vi "R5SetCalibrateConstant.vi"(0 "Signal":string, 1 "LabVIEW Web Service Request":refnum<class "Web Request.lvclass">, 5 "Write":bool, 7 "ReactorNo":i32=1, 9 "Slope":dbl, 11 "Intercept":dbl) -> (4 "Status":string[](array[string]), 8 "OldSlope":dbl, 10 "OldIntercept":dbl, 14 "NewIntercept":dbl, 15 "NewSlope":dbl)   [LabVIEW 2016]
uses:
  <vilib>/wsapi/Web Request.lvclass
  <resource>/objmgr/ni.var.rc
panel:
  in  "cRIONo":i32=1
  # "Use the Web Service Request input terminal to call the VIs on the Web Services palette. Do not remove it from the connector pane unless you don't need access to the palette."
  # "Each additional control wired to the connector pane will be available as an input in the URL. To include an indicator in terminal-mode output (the default setting), it must also be wired to the connector pane."
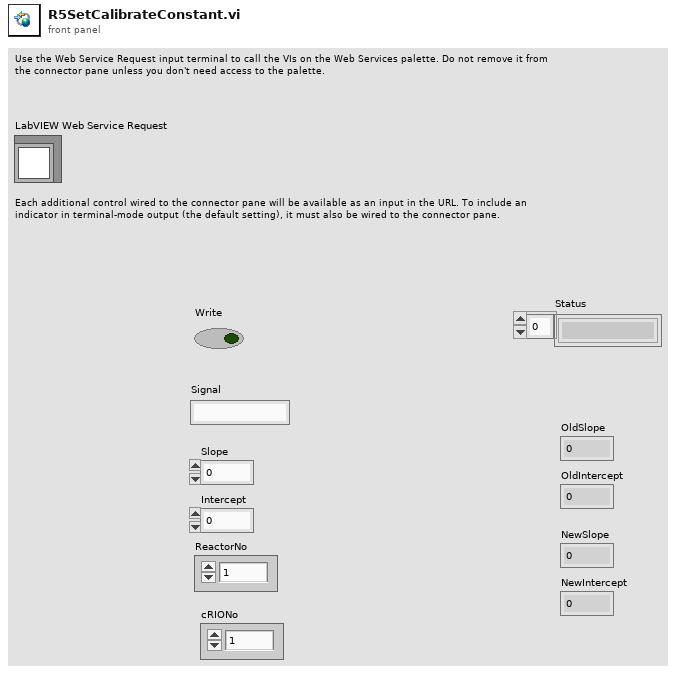
[diagram p1: front panel]
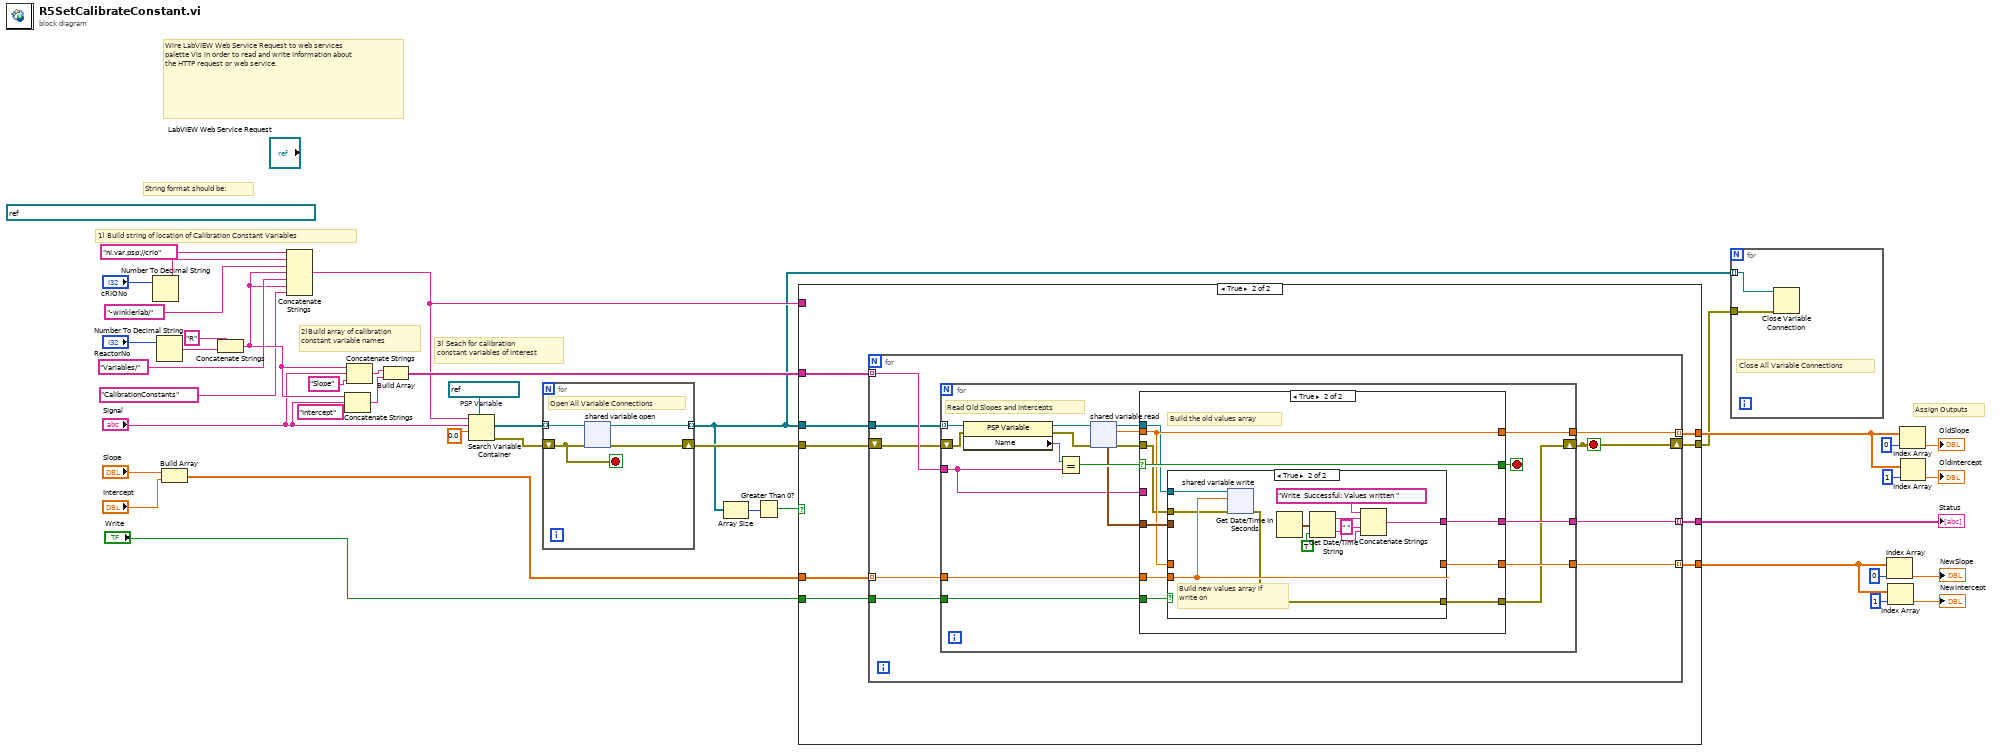
[diagram p0: block diagram]
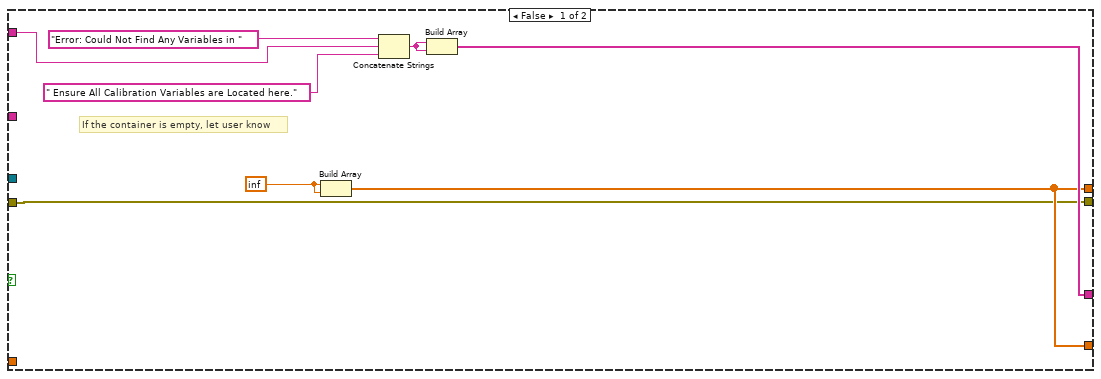
[diagram p2: hidden frame]
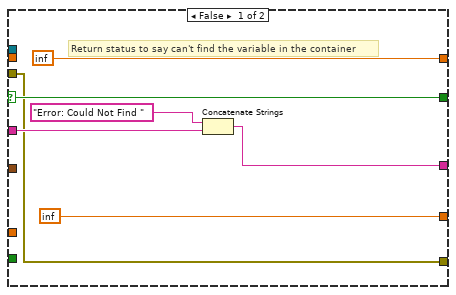
[diagram p3: hidden frame]
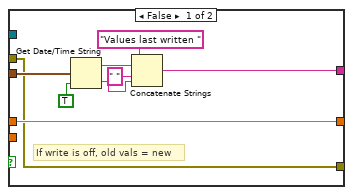
[diagram p4: hidden frame]
diagram:
  w25 = refnum<k21> refnum  # PSP Variable
  (unwired) refnum<k21> "ni.var.psp://crio1-winklerlab/R1Variables/R1CalibrationConstants" ("container refnum in")
  # "Assign Outputs"
  # "3) Seach for calibration \nconstant variables of interest"
  # "2)Build array of calibration \nconstant variable names"
  # "1) Build string of location of Calibration Constant Variables"
  # "String format should be:"
  # "Wire LabVIEW Web Service Request to web services palette VIs in order to read and write information about the HTTP request or web service."
  n1 = Number To Decimal String(number="cRIONo") -> (decimal integer string=w30:string)  [unwired: 1 in]
  n2 = Number To Decimal String(number="ReactorNo") -> (decimal integer string=w38:string)  [unwired: 1 in]
  n3 = Build Array("Slope", "Intercept") -> (w23:dbl[])
  n4 = Concatenate Strings("R" ("string"), w38) -> (w27:string)
  n5 = Concatenate Strings("ni.var.psp://crio" ("string"), w30, "-winklerlab/" ("string"), w27, "Variables/" ("string"), w27, "CalibrationConstants" ("string")) -> (w7:string)
  n6 = Concatenate Strings(w27, "Signal", "Intercept") -> (w36:string)
  n7 = Concatenate Strings(w27, "Signal", "Slope") -> (w37:string)
  n8 = Build Array(w37, w36) -> (w35:string[])
  n9 = Search Variable Container(7:w25, 9:0.0, 10:"Signal", 11:w7) -> (0:w11:errorcluster, 2:w12:refnum<k21>[])  [unwired: 2 in, 1 out]
  n10 = for {
    tunnel: w12 -> [w45] mode=indexing
    shift-right: [w44] -> w10
    shift-left: w11 -> [w42]
    tunnel: [w43] -> w1 mode=indexing
    stop <- w42 stop-if-true
    # "Open All Variable Connections"
    n11 = shared-variable-open(w45, w42) -> (w43:refnum<k21>, w44:errorcluster)  [unwired: 1 in]
  }
  n12 = Array Size(array=w1) -> (size(s)=w9:i32)
  n13 = Greater Than 0?(x=w9) -> (x > 0?=w8:bool)
  n14 = case shown="True" w8 {
    tunnel: w35 -> [_ w62]
    tunnel: "Write" -> [_ w61]
    tunnel: w23 -> [_ w60]
    tunnel: [w48 w59] -> w20
    tunnel: [w48 w58] -> w15
    tunnel: [w49 w57] -> w6
    tunnel: w1 -> [_ w56]
    tunnel: w10 -> [w46 w54]
    tunnel: w7 -> [w52 _]
    tunnel: [w46 w55] -> w2
    frame False {
      w50 = inf
      # "If the container is empty, let user know"
      n15 = Build Array(w50, w50) -> (w48:dbl[])
      n16 = Concatenate Strings("Error: Could Not Find Any Variables in " ("string"), w52, " Ensure All Calibration Variables are Located here." ("string")) -> (w51:string)
      n17 = Build Array(w51, w51) -> (w49:string[])
    }
    frame True {
      n18 = for {
        tunnel: w62 -> [w71] mode=indexing
        tunnel: w56 -> [w65]
        tunnel: w61 -> [w70]
        tunnel: w60 -> [w67] mode=indexing
        tunnel: [w69] -> w59 mode=indexing
        tunnel: [w68] -> w58 mode=indexing
        tunnel: [w66] -> w57 mode=indexing
        shift-right: [w64] -> w55
        shift-left: w54 -> [w63]
        stop <- w64 stop-if-true
        n19 = for {
          tunnel: w65 -> [w77] mode=indexing
          tunnel: w71 -> [w80]
          tunnel: w70 -> [w83]
          tunnel: [w85] -> w69
          tunnel: [w82] -> w68
          tunnel: [w81] -> w66
          tunnel: w67 -> [w79]
          shift-right: [w72] -> w64
          shift-left: w63 -> [w75]
          stop <- w78 stop-if-true
          # "Read Old Slopes and Intercepts"
          n20 = property class="PSP Variable"(reference=w77, error in=w75) -> (reference out=w76:refnum<k21>, error out=w74:errorcluster, "Name"=w73:string)
          n21 = Equal?(x=w73, y=w80) -> (x = y?=w86:bool)
          n22 = shared-variable-read(w76, w74) -> (w89:refnum<k21>, w87:errorcluster, w88:dbl, w84:timestamp)
          n23 = case shown="True" w86 {
            selector: w86 -> [w96 w106]
            tunnel: w89 -> [_ w99]
            tunnel: w88 -> [_ w103]
            tunnel: w87 -> [w90 w98]
            tunnel: [w96 w106] -> w78
            tunnel: [inf w103] -> w85
            tunnel: w84 -> [_ w105]
            tunnel: w83 -> [_ w104]
            tunnel: [inf w102] -> w82
            tunnel: [w92 w101] -> w81
            tunnel: w80 -> [w93 _]
            tunnel: w79 -> [_ w100]
            tunnel: [w90 w97] -> w72
            frame False {
              # "Return status to say can't find the variable in the container"
              n24 = Concatenate Strings("Error: Could Not Find " ("string"), w93) -> (w92:string)
            }
            frame True {
              # "Build the old values array"
              n25 = case shown="True" w104 {
                tunnel: w105 -> [w114 _]
                tunnel: [w110 w120] -> w101
                tunnel: w103 -> [w108 _]
                tunnel: [w108 w118] -> w102
                tunnel: w100 -> [_ w118]
                tunnel: w99 -> [_ w119]
                tunnel: w98 -> [w107 w117]
                tunnel: [w107 w116] -> w97
                frame False {
                  # "If write is off, old vals = new"
                  n26 = Get Date/Time String(seconds (now)=w114, want seconds? (F)=TRUE) -> (date string=w113:string, time string=w111:string)  [unwired: 1 in]
                  n27 = Concatenate Strings("Values last written " ("string"), w113, " " ("string"), w111) -> (w110:string)
                }
                frame True {
                  # "Build new values array if \nwrite on"
                  n28 = shared-variable-write(w119, w117, w118) -> (w116:errorcluster)  [unwired: 1 out]
                  n29 = Get Date/Time In Seconds() -> (seconds since 1Jan1904=w121:timestamp)
                  n30 = Get Date/Time String(seconds (now)=w121, want seconds? (F)=TRUE) -> (date string=w123:string, time string=w125:string)  [unwired: 1 in]
                  n31 = Concatenate Strings("Write  Successful: Values written " ("string"), w123, " " ("string"), w125) -> (w120:string)
                }
              }
            }
          }
        }
      }
    }
  }
  "Status" <- w6
  n32 = for {
    tunnel: w2 -> [w128]
    tunnel: w1 -> [w127] mode=indexing
    # "Close All Variable Connections"
    n33 = Close Variable Connection(8:w128, 11:w127) -> ()  [unwired: 1 out]
  }
  n34 = Index Array(array=w15, index=0) -> (element=→"NewSlope":dbl)
  n35 = Index Array(array=w15, index=1) -> (element=→"NewIntercept":dbl)
  n36 = Index Array(array=w20, index=0) -> (element=→"OldSlope":dbl)
  n37 = Index Array(array=w20, index=1) -> (element=→"OldIntercept":dbl)
